vi "read_ctab.vi"(5 "Array 2":cluster{"Uin":dbl[][]}[](array[cluster]), 7 "Path":path) -> (1 "Array":cluster{"Uin":dbl[][]}[](array[cluster]))   [LabVIEW 2010]
uses:
  <vilib>/Utility/xml.llb/Read From XML File(string).vi
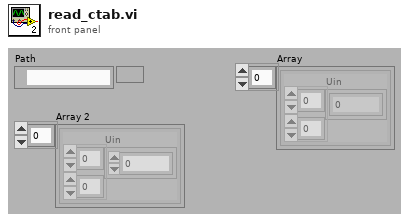
[diagram p1: front panel]
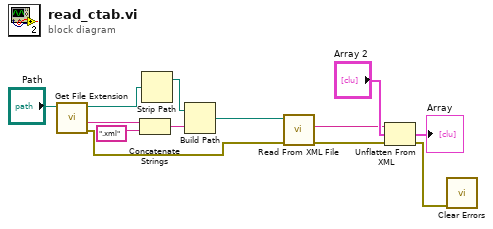
[diagram p0: block diagram]
diagram:
  n1 = call <vilib>:"Get File Extension.vi"("file"="Path") -> ("error out"=w2:errorcluster, "filename without extension"=w5:string, "dup file"=w7:path)  [unwired: 7 in, 1 out]
  n2 = Concatenate Strings(w5, ".xml" ("string")) -> (w3:string)
  n3 = Strip Path(path=w7) -> (stripped path=w6:path)  [unwired: 1 out]
  n4 = Build Path(base path=w6, name or relative path=w3) -> (appended path=w8:path)
  n5 = call-poly <vilib>:"Read From XML File.vi"("error in (no error)"=w2, "XML File Path"=w8) -> ("error out"=w11:errorcluster, "XML Elements"=w9:string)  [unwired: 7 in, 1 out]
  n6 = Unflatten From XML(xml string=w9, type="Array 2", error in (no error)=w11) -> (value=→"Array":cluster{"Uin":dbl[][]}[], error out=w1:errorcluster)
  n7 = call <vilib>:"Clear Errors.vi"("error in (no error)"=w1) -> ()  [unwired: 6 in, 1 out]
